vi "Write Speed.vi"   [LabVIEW 2013, in "APU.lvclass"]
uses:
  APU/APU.lvclass
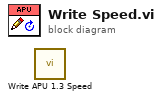
[diagram p0: block diagram]
diagram:
  n1 = call "Write APU 1.3 Speed.vi"() -> ()  [unwired: 10 in, 2 out]
